vi "SetThresholds.vi"(8 "ErrorIn":errorcluster, 9 "Set default thresholds? [F]":bool) -> (0 "ErrorOut":errorcluster={"status"=TRUE, "code"=1073, "source"="Invoke Node in SetThresholds.vi->master.vi->main.vi\n<APPEND>\nMethod Name: <b>Default Values:Make Current Default</b>"})   [LabVIEW 2019]
uses:
  MobileAnalyzer/mainVIs/utilities/FGVAction.ctl
  MobileAnalyzer/mainVIs/analyzeAccelerationDataVIs/calculateFaultIndicatorsVIs/Thresholds.ctl
  MobileAnalyzer/mainVIs/analyzeAccelerationDataVIs/calculateFaultIndicatorsVIs/FaultParameter.ctl
panel:
  in  "RMS":dbl
  in  "Czêstotliwoœci i progi":dbl[][](array[numeric])=[[50.0, 0.0]]
  in  "Kurtoza":dbl
  in  "Close":bool
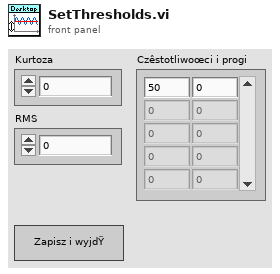
[diagram p1: front panel]
types:
  T1 = typedef "FGVAction.ctl" = enum16{"Read", "Write"}
  T2 = typedef "FaultParameter.ctl" = enum16{"Kurtosis", "RMS"}
  T3 = typedef "Thresholds.ctl" = cluster{"Parameters labels":T2[], "Parameters thresholds":dbl[], "Freqs and thresholds":dbl[][]}
  T4 = typedef "DesktopAppSettings.ctl" = cluster{"MobileAnalyzer IP":string, "Network Stream Timeout Code":i32, "Endpoint Destroyed Code":i32, "Save to file?":bool, "All threads":T5[], "Fault Thresholds":T3}
  T5 = typedef "Thread.ctl" = enum16{"GUI", "communicateWithAnalyzer", "saveDataToTDMS"}
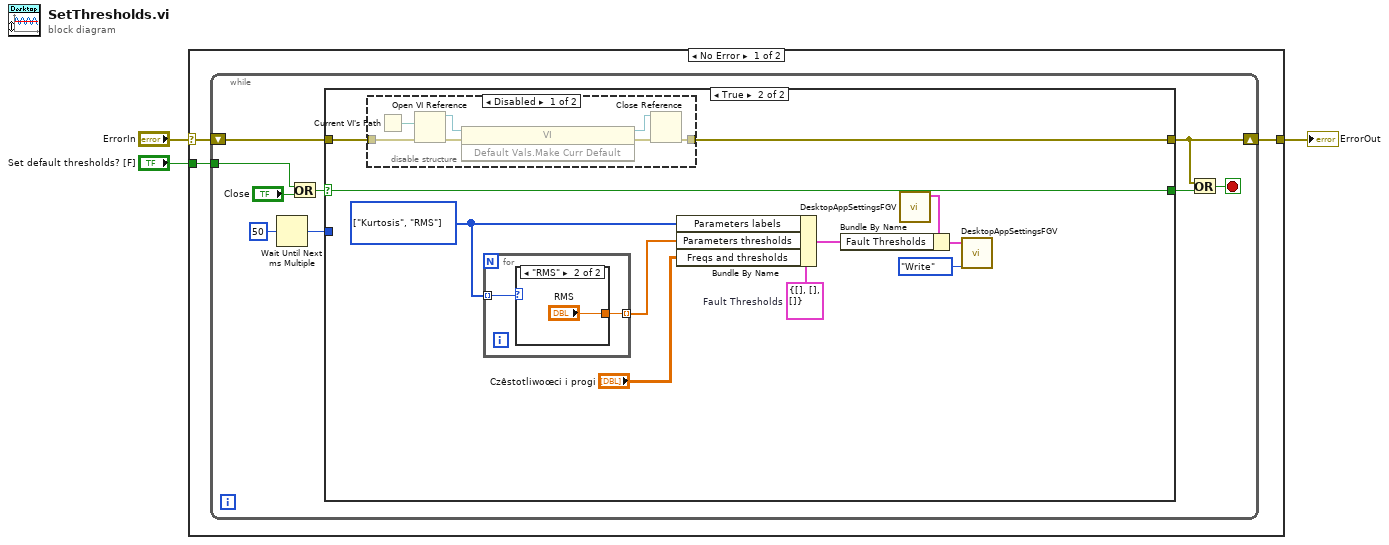
[diagram p0: block diagram]
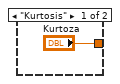
[diagram p3: hidden frame]
diagram:
  n1 = case shown="No Error" "ErrorIn" {
    selector: "ErrorIn" -> [w6 w40]
    tunnel: [w5 w40] -> w2
    tunnel: "Set default thresholds? [F]" -> [w4 _]
    frame No Error {
      n2 = while {
        shift-right: [w9] -> w5
        shift-left: w6 -> [w10]
        tunnel: w4 -> [w7]
        stop <- w15 stop-if-true
        n3 = Wait Until Next ms Multiple(millisecond multiple=u32 50) -> (millisecond timer value=w12:u32)
        n4 = Or(x=w7, y="Close") -> (x .or. y?=w8:bool)
        n5 = case shown="True" w8 {
          selector: w8 -> [_ w27]
          tunnel: w12 -> [_ _]
          tunnel: [_ w27] -> w11
          tunnel: w10 -> [w16 w22]
          tunnel: [w16 w21] -> w9
          frame False {
          }
          frame True {
            w19 = T2[] [enum."Kurtosis", enum."RMS"] items=["Kurtosis", "RMS"]
            w20 = T3 {"Parameters labels"=[], "Parameters thresholds"=[], "Freqs and thresholds"=[]}  # Fault Thresholds
            n6 = disable-structure shown="Disabled" {
              disable-tunnel: w22 -> [w33 w39]
              disable-tunnel: [w32 w39] -> w21
              frame Disabled {
                n7 = Current VI's Path() -> (path=w34:path)
                n8 = Open VI Reference(vi path=w34, error in (no error)=w33) -> (vi reference=w36:refnum<vi>, error out=w35:errorcluster)  [unwired: 4 in]
                n9 = invoke class="VI" method="Default Vals.Make Curr Default"(reference=w36, error in=w35) -> (reference out=w38:refnum<vi>, error out=w37:errorcluster)  [unwired: 1 in, 1 out]
                n10 = Close Reference(reference=w38, error in (no error)=w37) -> (error out=w32:errorcluster)
              }
              frame Enabled {
              }
            }
            n11 = for {
              tunnel: w19 -> [w29] mode=indexing
              tunnel: [w28] -> w18 mode=indexing
              n12 = case shown="\"RMS\"" w29 {
                tunnel: ["Kurtoza" "RMS"] -> w28
                frame "Kurtosis" {
                }
                frame "RMS" {
                }
              }
            }
            n13 = Bundle By Name(cluster=w20, "Parameters labels"=w19, "Parameters thresholds"=w18, "Freqs and thresholds"="Czêstotliwoœci i progi") -> (w26:T3)
            n14 = call "DesktopAppSettingsFGV.vi"() -> ("DesktopAppSettingsOut"=w24:T4)  [unwired: 11 in]
            n15 = Bundle By Name(cluster=w24, "Fault Thresholds"=w26) -> (w23:T4)
            n16 = call "DesktopAppSettingsFGV.vi"("FGVAction (Read)"=FGVAction."Write", "DesktopAppSettingsIn"=w23) -> ()  [unwired: 9 in, 1 out]
          }
        }
        n17 = Or(x=w9, y=w11) -> (x .or. y?=w15:bool)
      }
    }
    frame Error {
    }
  }
  "ErrorOut" <- w2
